vi "PLExcimerPan.vi"(8 "error in (no error)":errorcluster caption="entrée d'erreur (pas d'erreur)", 11 "EGG5210.lvclass":refnum<class "EGG5210.lvclass">) -> (0 "error out":errorcluster caption="sortie d'erreur", 3 "EGG5210.lvclass Out":refnum<class "EGG5210.lvclass">)   [LabVIEW 2010, in "EGG5210.lvclass"]
uses:
  EGG5210.lvclass
  <userlib>/EG_G 5210 LIA/TrigMode.ctl
  BaseDevice/BaseDevice.lvclass
  <userlib>/EG_G 5210 LIA/ReadFunctions.ctl
  EGG5210.lvclass/EGG5210.ctl
panel:
  out "ADC Value":dbl
  in  "ADC Delay (ms)":u32=50 min=1 step=1
  in  "Trigger Mode":T1=2 items=["Reference", "External", "Asynchronous", "Ratio", "8F"]
  in  "Laser Trigg.":bool
  out "Min.Delay (ms)":u32
  in  "Acq":bool
  in  "Excitation (Hz)":dbl=8.0 min=0.5 max=100000.0 step=0.01
  in  "Boxcar Aver. #":u32=1 min=1 step=1
  in  "ADC Average #":u32=1 min=1 step=1
  in  "Stop":bool
  out "Init Program":bool
  # "PL Excimer Settings"
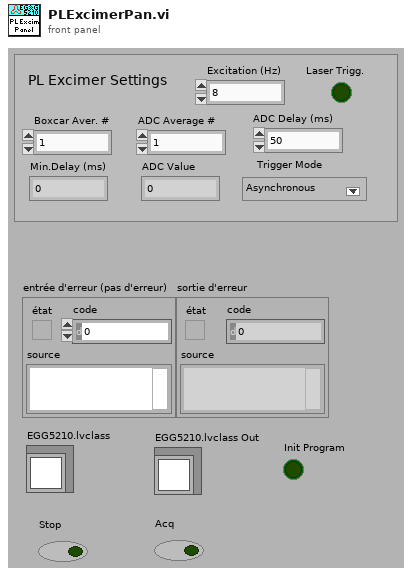
[diagram p1: front panel]
types:
  T1 = typedef "TrigMode.ctl" = u16
  T2 = typedef "ReadFunctions.ctl" = enum16{"Sensitivity", "Vernier Mode", "Main Filter", "Filter Mode", "Line Filter", "Ref Source", "Ref Mode", "Ref Phase", "Ref Frequency", "Output Filter", "Time Constant", "Dyn Reserve", "X Offset", "Y Offset", "Expand Mode", "Int Oscillator", "Oscillator Freq", "All params", "Overload Byte", "Trigger Mode", "Error"}
  T3 = enum8{"Enabled", "Disabled", "Disabled and Grayed Out"}
  T4 = typedef "LockInPar.ctl" = cluster{"Sensitivity":u16, "Vernier Mode":bool, "Vernier Value":i32, "Main Filter":u16, "Filter Freq (Hz)":dbl, "Filter Mode":u16, " Line Notch":u16, "Reference":u16, "Reference Mode":u16, "Ref Phase (°)":dbl, "Ref Freq (Hz)":dbl, "Output Filter":u16, "Time Constant":u16, "Dynamic Res.":u16, "X Offset":bool, "X Offset Val %":dbl, "Y Offset":bool, "Y Offset Val %":dbl, "Expand":bool, "Osc Amp. (mV rms)":i32, "Int Osc (Hz)":dbl, "Trigger Mode":T1, "Input Mode":u16, "Ovld Source":u16}
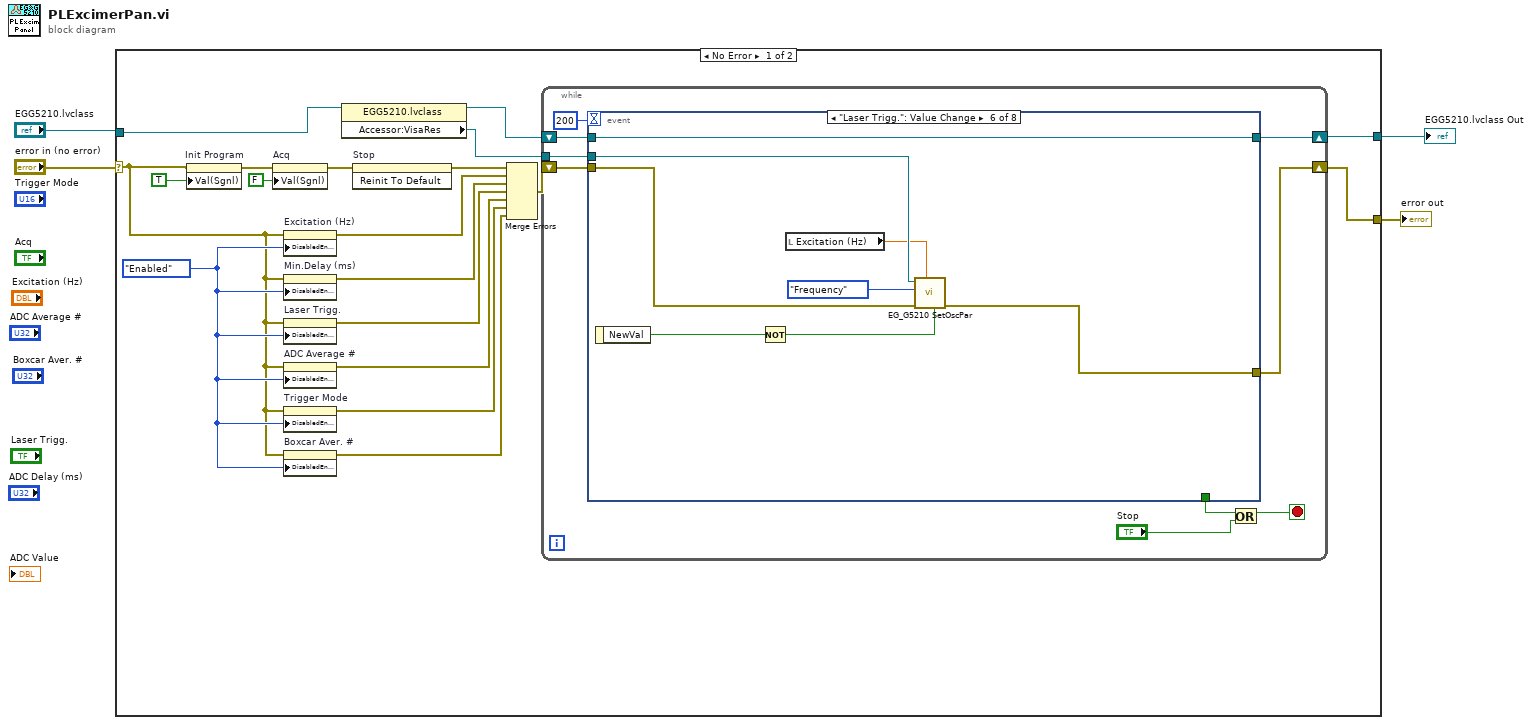
[diagram p0: block diagram]
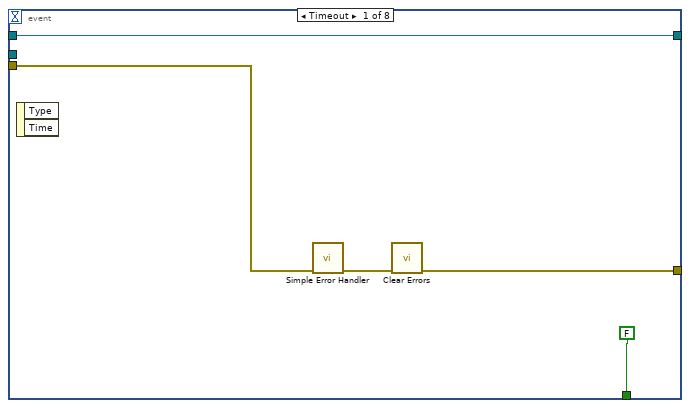
[diagram p2: hidden frame]
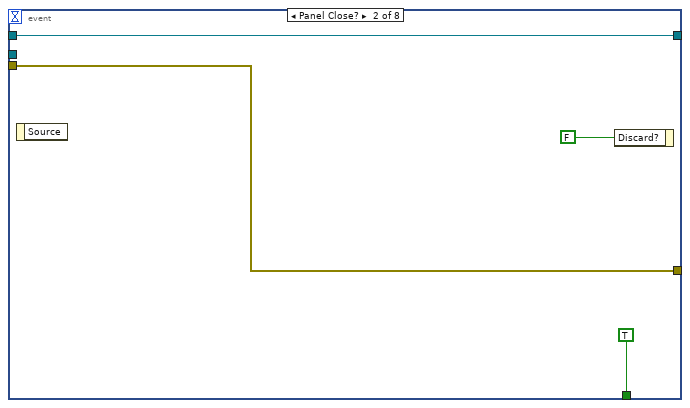
[diagram p3: hidden frame]
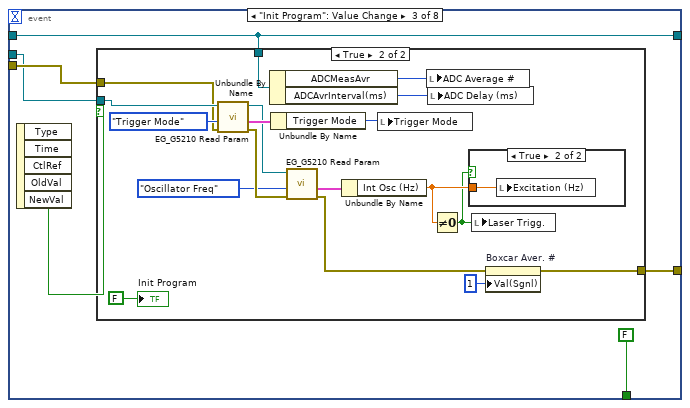
[diagram p4: hidden frame]
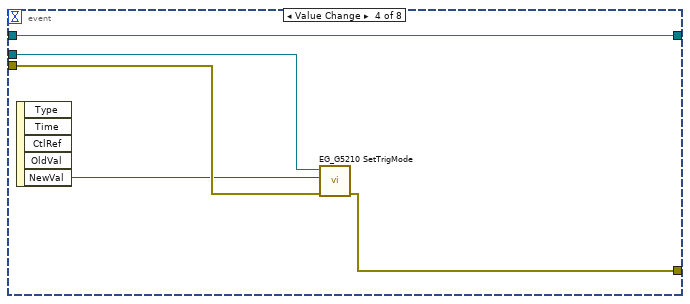
[diagram p7: hidden frame]
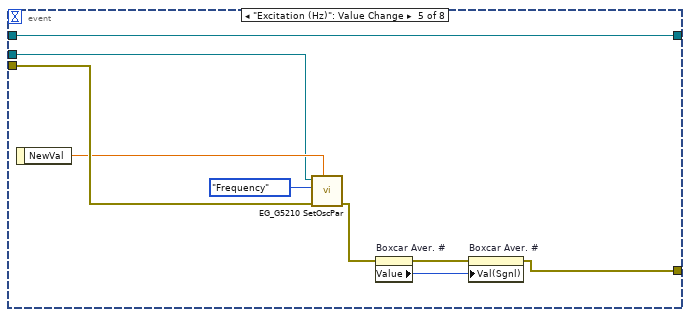
[diagram p8: hidden frame]
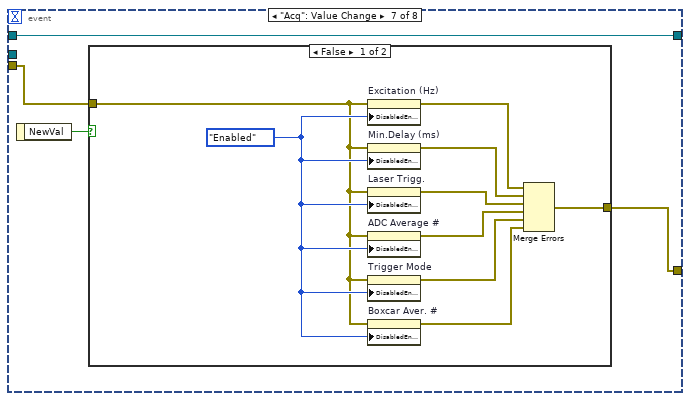
[diagram p9: hidden frame]
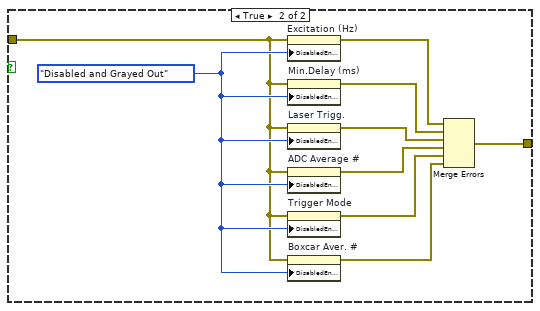
[diagram p10: hidden frame]
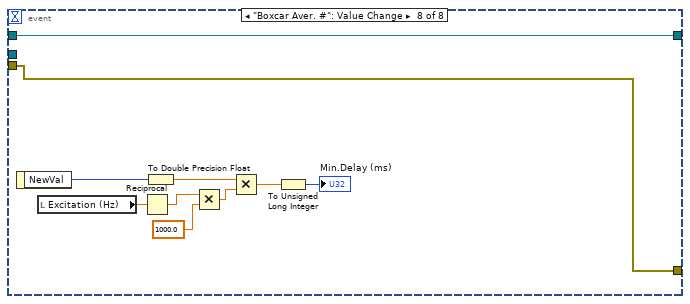
[diagram p11: hidden frame]
diagram:
  n1 = case shown="No Error" "error in (no error)" {
    selector: "error in (no error)" -> [w12 w123]
    tunnel: [w23 w123] -> w3
    tunnel: "EGG5210.lvclass" -> [w20 w122]
    tunnel: [w22 w122] -> w2
    frame No Error {
      w13 = T3."Enabled" ("Désactivé")
      n2 = property on="Init Program" class="Bool (strict)"(error in=w12, "Val(Sgnl)"=TRUE ("Valeur (Signalisation)")) -> (error out=w17:errorcluster)  [unwired: 1 in, 1 out]
      n3 = property on="Acq" class="Bool (strict)"(error in=w17, "Val(Sgnl)"=FALSE ("Valeur (Signalisation)")) -> (error out=w16:errorcluster)  [unwired: 1 in, 1 out]
      n4 = property on="Excitation (Hz)" class="DigNum (strict)"(error in=w12, "DisabledEnum"=w13) -> (error out=w10:errorcluster)  [unwired: 1 in, 1 out]
      n5 = property on="Min.Delay (ms)" class="DigNum (strict)"(error in=w12, "DisabledEnum"=w13) -> (error out=w9:errorcluster)  [unwired: 1 in, 1 out]
      n6 = property on="Laser Trigg." class="Bool (strict)"(error in=w12, "DisabledEnum"=w13) -> (error out=w8:errorcluster)  [unwired: 1 in, 1 out]
      n7 = property on="ADC Average #" class="DigNum (strict)"(error in=w12, "DisabledEnum"=w13) -> (error out=w7:errorcluster)  [unwired: 1 in, 1 out]
      n8 = property on="Trigger Mode" class="Ring (strict)"(error in=w12, "DisabledEnum"=w13) -> (error out=w6:errorcluster)  [unwired: 1 in, 1 out]
      n9 = property on="Boxcar Aver. #" class="DigNum (strict)"(error in=w12, "DisabledEnum"=w13) -> (error out=w5:errorcluster)  [unwired: 1 in, 1 out]
      n10 = property class="EGG5210.lvclass"(reference=w20) -> (reference out=w19:refnum<class "EGG5210.lvclass">, "Accessor:VisaRes"=w18:refnum<visa-resource-name>)  [unwired: 1 in, 1 out]
      n11 = invoke on="Stop" class="Bool (strict)" method="Reinit To Default"(error in=w16) -> (error out=w21:errorcluster)  [unwired: 2 in, 2 out]
      n12 = Merge Errors(w21, w10, w9, w8, w7, w6, w5) -> (w11:errorcluster)
      n13 = while {
        shift-right: [w30] -> w23
        shift-left: w11 -> [w31]
        shift-right: [w27] -> w22
        shift-left: w19 -> [w29]
        tunnel: w18 -> [w24]
        stop <- w26 stop-if-true
        n14 = event shown="[5] \"Laser Trigg.\": Value Change" {
          selector: _ -> [_ _ _ _ _ _ _ _]
          dyn-events: _ -> [_ _ _ _ _ _ _ _]
          timeout: 200 -> [_ _ _ _ _ _ _ _]
          tunnel: w31 -> [w35 w39 w46 w71 w80 w88 w91 w112]
          tunnel: [w33 w39 w45 w69 w76 w87 w90 w112] -> w30
          tunnel: w29 -> [w36 w38 w42 w68 w81 w89 w92 w118]
          tunnel: [FALSE TRUE FALSE _ _ _ _ _] -> w28
          tunnel: [w36 w38 w42 w68 w81 w89 w92 w118] -> w27
          tunnel: w24 -> [_ _ w43 w72 w78 w86 _ _]
          event Timeout {
            n15 = event-data() -> ()  [unwired: 1 in, 2 out]
            n16 = call <vilib>:"Simple Error Handler.vi"("error in (no error)"=w35) -> ("error out"=w34:errorcluster)  [unwired: 4 in, 4 out]
            n17 = call <vilib>:"Clear Errors.vi"("error in (no error)"=w34) -> ("error out"=w33:errorcluster)  [unwired: 6 in]
          }
          event Panel Close? {
            n18 = event-data() -> ()  [unwired: 1 in, 1 out]
            n19 = event-data("Discard?"=FALSE ("Rejeter ?")) -> ()  [unwired: 1 in, 1 out]
          }
          event "Init Program": Value Change {
            n20 = event-data() -> ("NewVal"=w47:bool)  [unwired: 1 in, 4 out]
            n21 = case shown="True" w47 {
              tunnel: w46 -> [w48 w61]
              tunnel: [w48 w50] -> w45
              tunnel: w43 -> [_ w62]
              tunnel: w42 -> [_ w54]
              frame False {
              }
              frame True {
                n22 = call <userlib>:"EG_G5210 Read Param.vi"("error in (no error)"=w61, "Énum"=ReadFunctions."Trigger Mode", "Ressource VISA"=w62) -> ("error out"=w60:errorcluster, "LockInPar"=w64:T4, "Ressource VISA Out"=w59:refnum<visa-resource-name>)  [unwired: 5 in, 1 out]
                n23 = Unbundle By Name(w54) -> ("ADCMeasAvr"=w53:u32, "ADCAvrInterval(ms)"=w52:u32)
                n24 = Unbundle By Name(w64) -> ("Trigger Mode"=w63:T1)
                n25 = call <userlib>:"EG_G5210 Read Param.vi"("error in (no error)"=w60, "Énum"=ReadFunctions."Oscillator Freq", "Ressource VISA"=w59) -> ("error out"=w51:errorcluster, "LockInPar"=w57:T4)  [unwired: 5 in, 2 out]
                n26 = Unbundle By Name(w57) -> ("Int Osc (Hz)"=w56:dbl)
                n27 = local write "Trigger Mode"(w63) -> ()
                n28 = local write "ADC Average #"(w53) -> ()
                n29 = local write "ADC Delay (ms)"(w52) -> ()
                n30 = Not Equal To 0?(x=w56) -> (x != 0?=w55:bool)
                n31 = case shown="True" w55 {
                  tunnel: w56 -> [_ w67]
                  frame False {
                  }
                  frame True {
                    n32 = local write "Excitation (Hz)"(w67) -> ()
                  }
                }
                n33 = local write "Laser Trigg."(w55) -> ()
                n34 = property on="Boxcar Aver. #" class="DigNum (strict)"(error in=w51, "Val(Sgnl)"=u32 1 ("Valeur (Signalisation)")) -> (error out=w50:errorcluster)  [unwired: 1 in, 1 out]
                "Init Program" <- FALSE
              }
            }
          }
          event Value Change {
            n35 = event-data() -> ("NewVal"=w70:T1)  [unwired: 1 in, 4 out]
            n36 = call <userlib>:"EG_G5210 SetTrigMode.vi"("error in (no error)"=w71, "TrigMode"=w70, "Ressource VISA"=w72) -> ("error out"=w69:errorcluster)  [unwired: 7 in, 1 out]
          }
          event "Excitation (Hz)": Value Change {
            n37 = event-data() -> ("NewVal"=w79:dbl)  [unwired: 1 in]
            n38 = call <userlib>:"EG_G5210 SetOscPar.vi"("Frequency"=w79, "error in (no error)"=w80, "Énum"=enum16{"Amplitude", "Frequency"}."Frequency", "Ressource VISA"=w78) -> ("error out"=w74:errorcluster)  [unwired: 6 in, 1 out]
            n39 = property on="Boxcar Aver. #" class="DigNum (strict)"(error in=w74) -> (error out=w75:errorcluster, "Value"=w73:u32)  [unwired: 1 in, 1 out]
            n40 = property on="Boxcar Aver. #" class="DigNum (strict)"(error in=w75, "Val(Sgnl)"=w73) -> (error out=w76:errorcluster)  [unwired: 1 in, 1 out]
          }
          event "Laser Trigg.": Value Change {
            n41 = event-data() -> ("NewVal"=w84:bool)  [unwired: 1 in]
            n42 = Not(x=w84) -> (.not. x?=w82:bool)
            n43 = local read "Excitation (Hz)"() -> (w83:dbl)
            n44 = call <userlib>:"EG_G5210 SetOscPar.vi"("Disable Osc"=w82, "Frequency"=w83, "error in (no error)"=w88, "Énum"=enum16{"Amplitude", "Frequency"}."Frequency", "Ressource VISA"=w86) -> ("error out"=w87:errorcluster)  [unwired: 5 in, 1 out]
          }
          event "Acq": Value Change {
            n45 = event-data() -> ("NewVal"=w93:bool)  [unwired: 1 in]
            n46 = case shown="False" w93 {
              tunnel: w91 -> [w101 w110]
              tunnel: [w94 w103] -> w90
              frame False {
                w102 = T3."Enabled" ("Désactivé")
                n47 = property on="Excitation (Hz)" class="DigNum (strict)"(error in=w101, "DisabledEnum"=w102) -> (error out=w100:errorcluster)  [unwired: 1 in, 1 out]
                n48 = property on="Min.Delay (ms)" class="DigNum (strict)"(error in=w101, "DisabledEnum"=w102) -> (error out=w99:errorcluster)  [unwired: 1 in, 1 out]
                n49 = property on="Laser Trigg." class="Bool (strict)"(error in=w101, "DisabledEnum"=w102) -> (error out=w98:errorcluster)  [unwired: 1 in, 1 out]
                n50 = property on="ADC Average #" class="DigNum (strict)"(error in=w101, "DisabledEnum"=w102) -> (error out=w97:errorcluster)  [unwired: 1 in, 1 out]
                n51 = property on="Trigger Mode" class="Ring (strict)"(error in=w101, "DisabledEnum"=w102) -> (error out=w96:errorcluster)  [unwired: 1 in, 1 out]
                n52 = property on="Boxcar Aver. #" class="DigNum (strict)"(error in=w101, "DisabledEnum"=w102) -> (error out=w95:errorcluster)  [unwired: 1 in, 1 out]
                n53 = Merge Errors(w100, w99, w98, w97, w96, w95) -> (w94:errorcluster)
              }
              frame True {
                w111 = T3."Disabled and Grayed Out" ("Désactivé")
                n54 = property on="Excitation (Hz)" class="DigNum (strict)"(error in=w110, "DisabledEnum"=w111) -> (error out=w109:errorcluster)  [unwired: 1 in, 1 out]
                n55 = property on="Min.Delay (ms)" class="DigNum (strict)"(error in=w110, "DisabledEnum"=w111) -> (error out=w108:errorcluster)  [unwired: 1 in, 1 out]
                n56 = property on="Laser Trigg." class="Bool (strict)"(error in=w110, "DisabledEnum"=w111) -> (error out=w107:errorcluster)  [unwired: 1 in, 1 out]
                n57 = property on="ADC Average #" class="DigNum (strict)"(error in=w110, "DisabledEnum"=w111) -> (error out=w106:errorcluster)  [unwired: 1 in, 1 out]
                n58 = property on="Trigger Mode" class="Ring (strict)"(error in=w110, "DisabledEnum"=w111) -> (error out=w105:errorcluster)  [unwired: 1 in, 1 out]
                n59 = property on="Boxcar Aver. #" class="DigNum (strict)"(error in=w110, "DisabledEnum"=w111) -> (error out=w104:errorcluster)  [unwired: 1 in, 1 out]
                n60 = Merge Errors(w109, w108, w107, w106, w105, w104) -> (w103:errorcluster)
              }
            }
          }
          event "Boxcar Aver. #": Value Change {
            n61 = event-data() -> ("NewVal"=w121:u32)  [unwired: 1 in]
            n62 = local read "Excitation (Hz)"() -> (w120:dbl)
            n63 = Reciprocal(x=w120) -> (1/x=w115:dbl)
            n64 = To Double Precision Float(number=w121) -> (double precision float=w119:dbl)
            n65 = Multiply(x=w115, y=1000.0) -> (x*y=w116:dbl)
            n66 = Multiply(x=w119, y=w116) -> (x*y=w113:dbl)
            n67 = To Unsigned Long Integer(number=w113) -> (unsigned 32bit integer=→"Min.Delay (ms)":u32)
          }
        }
        n68 = Or(x=w28, y="Stop") -> (x .or. y?=w26:bool)
      }
    }
    frame Error {
    }
  }
  "error out" <- w3
  "EGG5210.lvclass Out" <- w2
